vi "Stokes_Num.vi"(9 "nu":dbl, 10 "omega":dbl[](array[numeric]), 11 "Do (mm)":dbl) -> (3 "Stokes number":dbl[](array[numeric]))   [LabVIEW 2012]
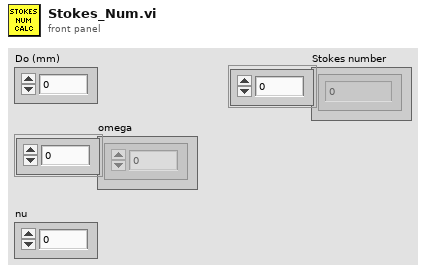
[diagram p1: front panel]
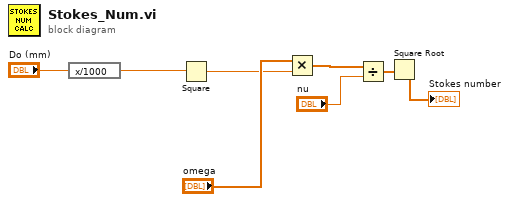
[diagram p0: block diagram]
diagram:
  n1 = expression code="x/1000"("Do (mm)") -> (w7:dbl)
  n2 = Square(x=w7) -> (x^2=w1:dbl)
  n3 = Multiply(x="omega", y=w1) -> (x*y=w2:dbl[])
  n4 = Divide(x=w2, y="nu") -> (x/y=w3:dbl[])
  n5 = Square Root(x=w3) -> (sqrt(x)=→"Stokes number":dbl[])
